vi "Traverse_Space_for new collision code.vi"(7 "Simulate/Run":T1=enum."Run VI", 9 "Show Panel?":bool, 10 "Traverse Setup":string) -> (3 "Error Comments":string)   [LabVIEW 2022 SP3]
doc: "This is an example of using features of the VI Server as a client. It shows how you might browse from one or more applications that may be exporting data from one or more data stations. \n\nThe example shows how to query a server for its list of exported VIs, how to get references to the VIs, and how call them with the Call By Reference function."
uses:
  Route mapping/Box_size.ctl
  Controls/ok_button.ctl
  Controls/User_Specific_mode.ctl
  Collision_Detection/Triangles/EnFlo specific/Collision Detection global.vi
  Globals/Constants_global.vi
  Globals/Trav_pos_global.vi
  Globals/Preference_global.vi
  Route mapping/Route_mapping_global.vi
panel:
  in  "Fixed Objects Name":u16(ring) items=["BeamCheck_Box_16500", "None"]
  out "Message":string
  in  "Probe Support":T2=[{"Max"=15001.0, "Min"=12000.0}, {"Max"=1000.0, "Min"=-1000.0}, {"Max"=700.0, "Min"=0.0}] {"Min" format="%#.1f"; "Max" format="%#.1f"}
  out "XYZ string":string
  out "XY string":string
  out "X string":string
  in  "X Component":u16(ring) items=["EnFlo_Trav1_X - Copy.stl", "EnFlo_Trav1_X.stl", "EnFlo_Trav1_X_original.stl", "Hello.stl", "None.stl"]
  in  "XYZ Component (Measurement Probe)":u16(ring) items=["None", "XYZ_20190131", "XYZ_20190918"]
  in  "XY Component (Traverse Boom)":u16(ring) items=["EnFlo_Trav1_XY.stl", "EnFlo_Trav1_XY_Long.stl", "EnFlo_Trav1_XY_Long_UW_laydown.stl", "EnFlo_Trav1_XY_Long_X400mm.stl", "EnFlo_Trav1_XY_Medium.stl", "EnFlo_Trav1_XY_Medium_FFID.stl", "EnFlo_Trav1_XY_Medium_UV_vertical.stl", "EnFlo_Trav1_XY_Medium_UW_laydown.stl", "None.stl"]
  in  "Model Name":u16(ring) items=["DIPLOS_array", "DIPLOS_array_0", "DIPLOS_array_45", "DSTL_Dapple_46", "Elysee", "Elysee_original", "Elysee_Source1", "Elysee_Source2", "Elysee_Source3", "MAGIC_1to500_Extra_8SE", "MAGIC_1to500_plus8", "MAGIC_1to500_plus8_fs", "MAGIC_London_Southbank_0_deg - Copy", "MAGIC_London_Southbank_0_deg _Case2", "MAGIC_London_Southbank_0_deg", "MAGIC_London_Southbank_0_deg_1to500", "MAGIC_London_Southbank_0_deg_1to500_without8SE", "MAGIC_London_Southbank_0_deg_21-08-19", "MAGIC_London_Southbank_0_deg_5_roofs", "MAGIC_London_Southbank_0_deg_ALL_roofs", "MAGIC_London_Southbank_0_deg_ALL_roofs_excl_bld12", "MAGIC_London_Southbank_0_deg_excl_12_and_150", "MAGIC_London_Southbank_0_deg_increasedHeights", "MAGIC_London_Southbank_0_deg_plus8", "MAGIC_London_Southbank_0_deg_plus8_bldg139roofblocks", "MAGIC_London_Southbank_0_deg_roofs", "MAGIC_London_Southbank_0_deg_roofs_3,8,10,49,60", "MAGIC_London_Southbank_0_deg_st8", "MAGIC_London_Southbank_VerMarco", "MAGIC_mic01_0_deg", "None", "Simple_C", "Simple_V", "Single_Cube_H240", "Single_Tall_Bldg"]
  in  "Traverse Name":u16(ring) items=["EnFlo_Stack", "EnFlo_Trav1", "EnFlo_Trav3", "EnFlo_Trav4", "EnFlo_Tunnel", "EnFlo_Turntable", "Laser_Disp_Scanner"]
  in  "Cancel Button":bool
  in  "OK":T3
  in  "Traverse Limits":T2=[{"Max"=15001.0, "Min"=12000.0}, {"Max"=1000.0, "Min"=-1000.0}, {"Max"=700.0, "Min"=0.0}] {"Min" format="%#.1f"; "Max" format="%#.1f"}
  # "Enter all coordinates assuming the Model Orientation is zero degrees"
  # "X                           Y                          Z"
  # "All geometry always reloaded after running this panel"
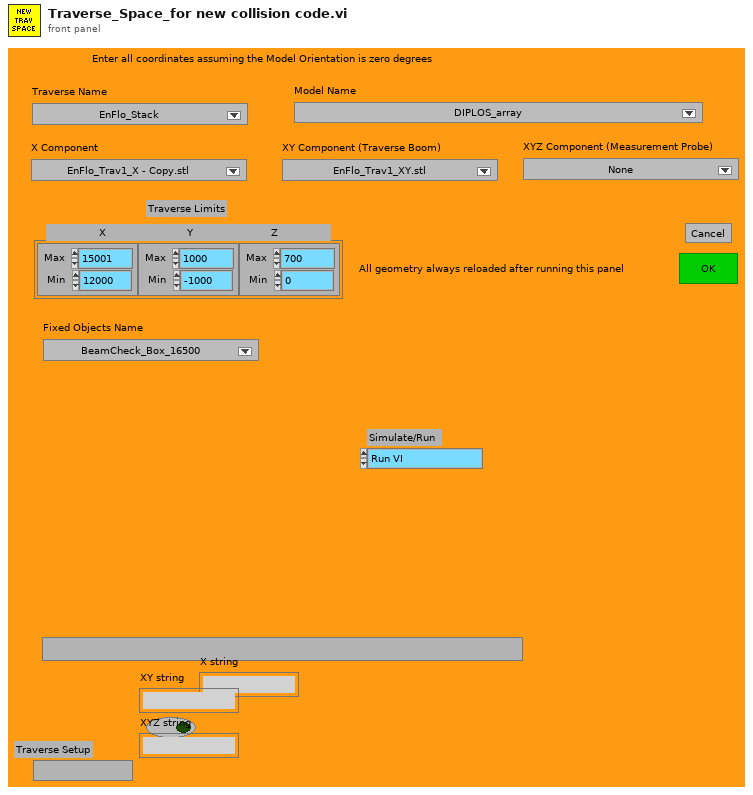
[diagram p1: front panel]
types:
  T1 = typedef "User_Specific_mode.ctl" = enum16{"Check VI only", "Run VI"}
  T2 = typedef "Box_size.ctl" = cluster{"Max":sgl, "Min":sgl}[]
  T3 = typedef "ok_button.ctl" = bool
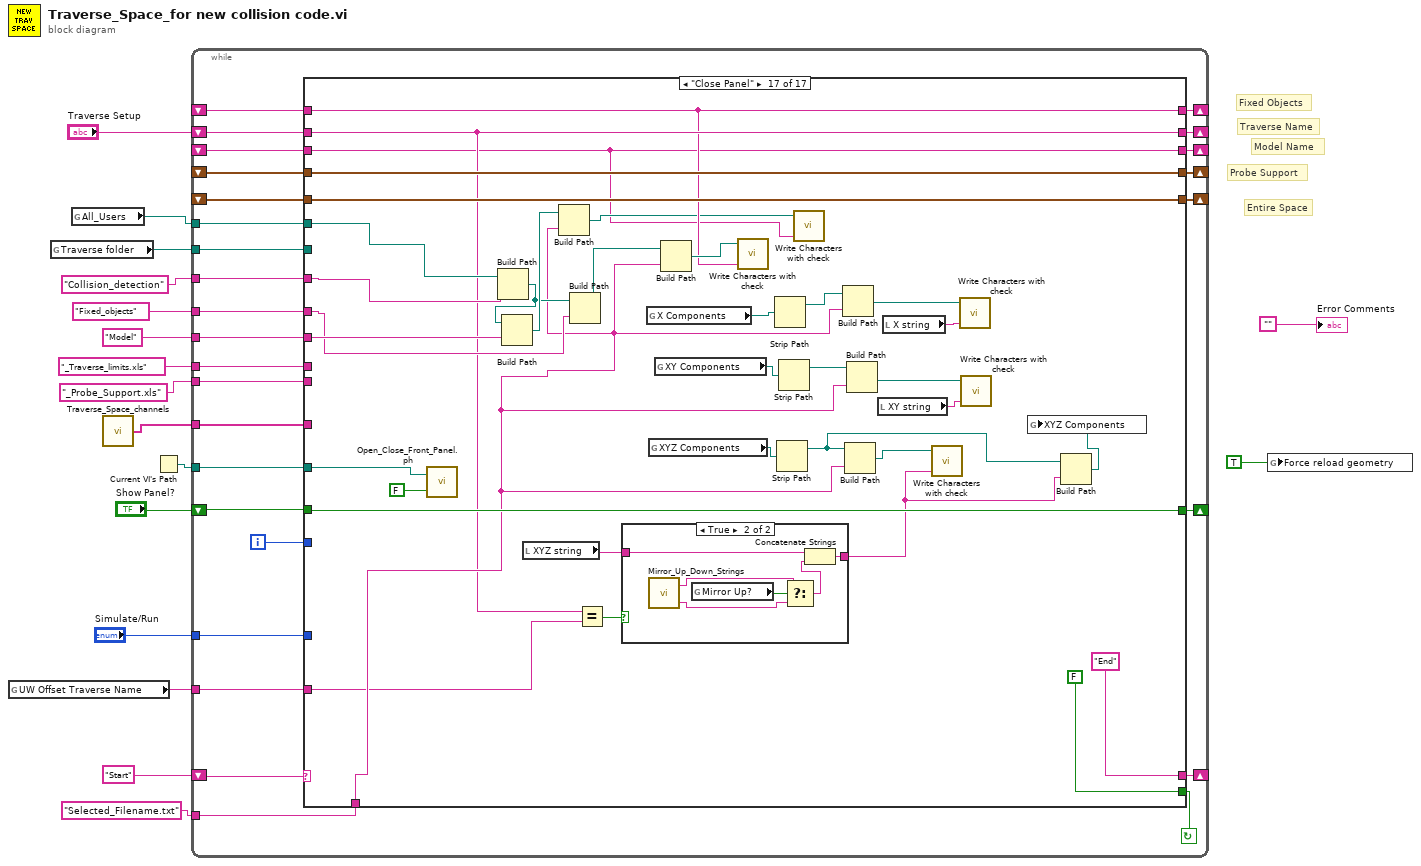
[diagram p0: block diagram]
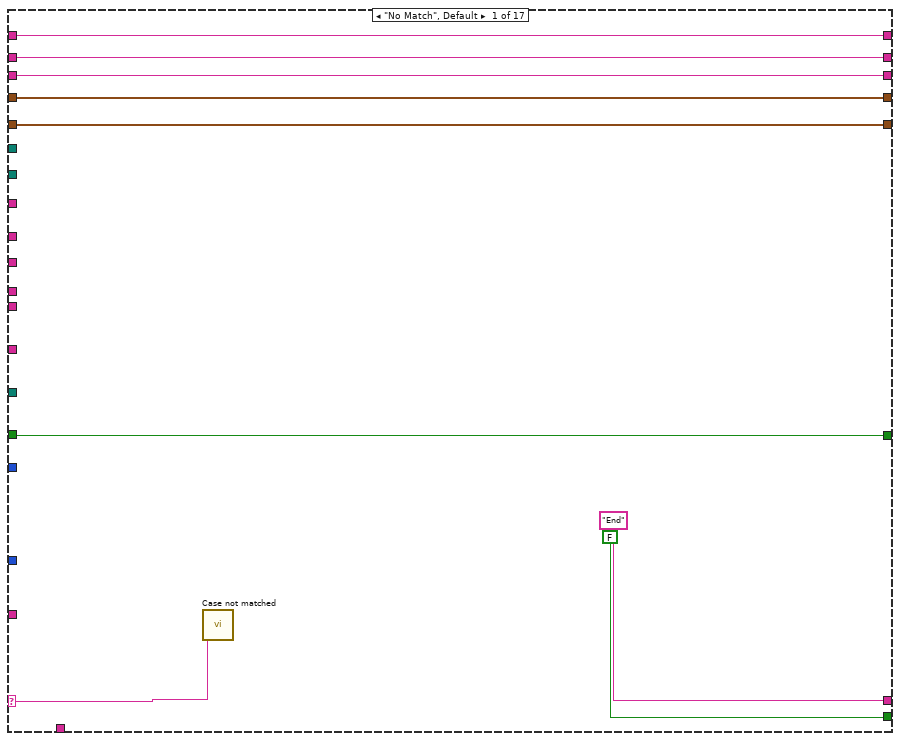
[diagram p2: hidden frame]
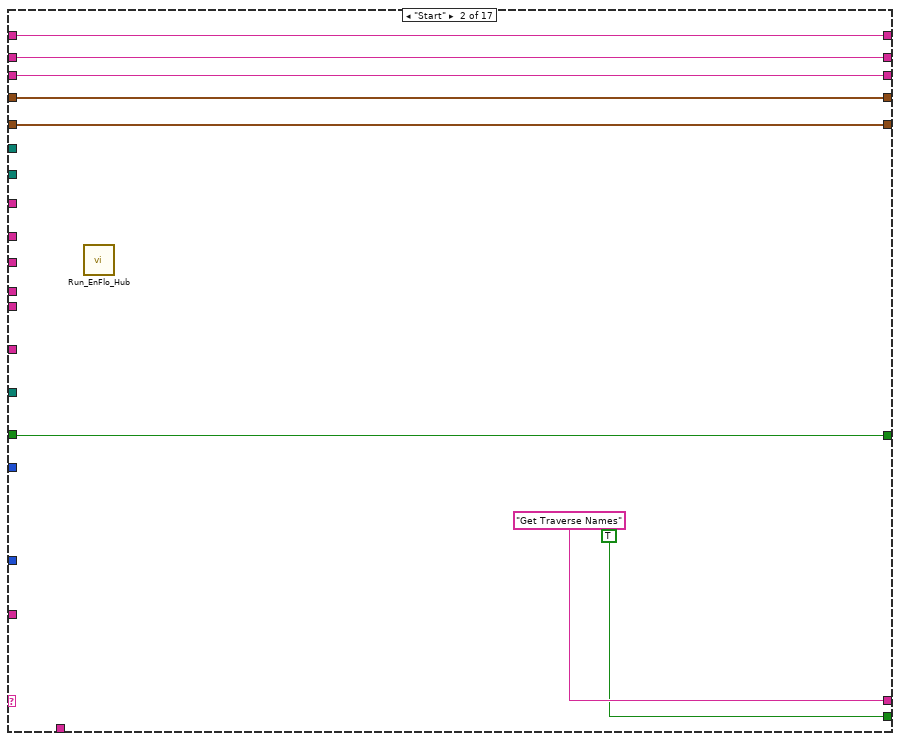
[diagram p3: hidden frame]
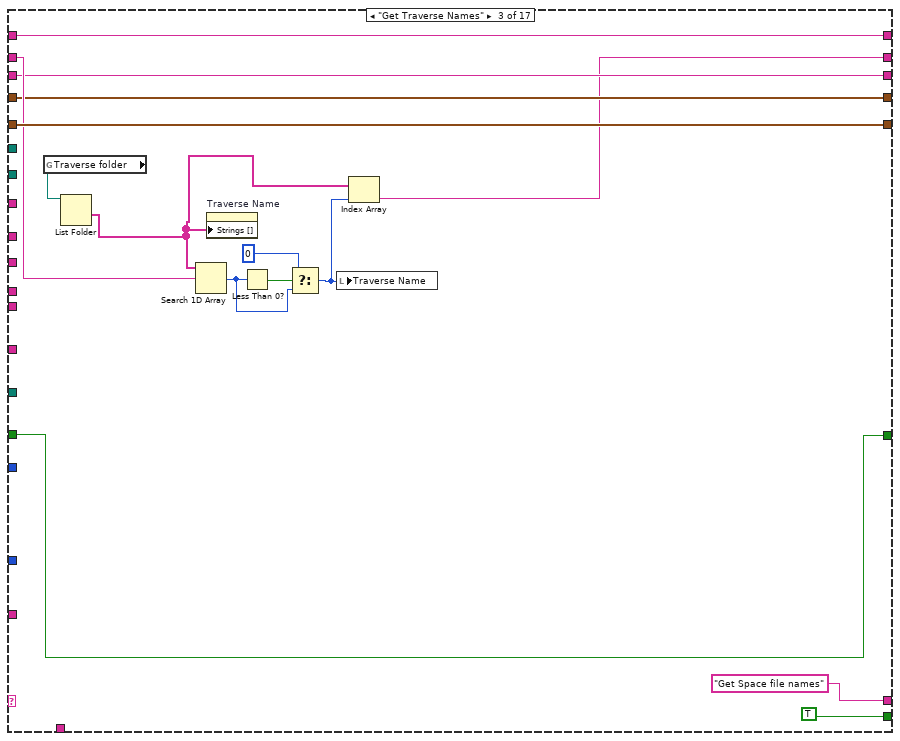
[diagram p4: hidden frame]
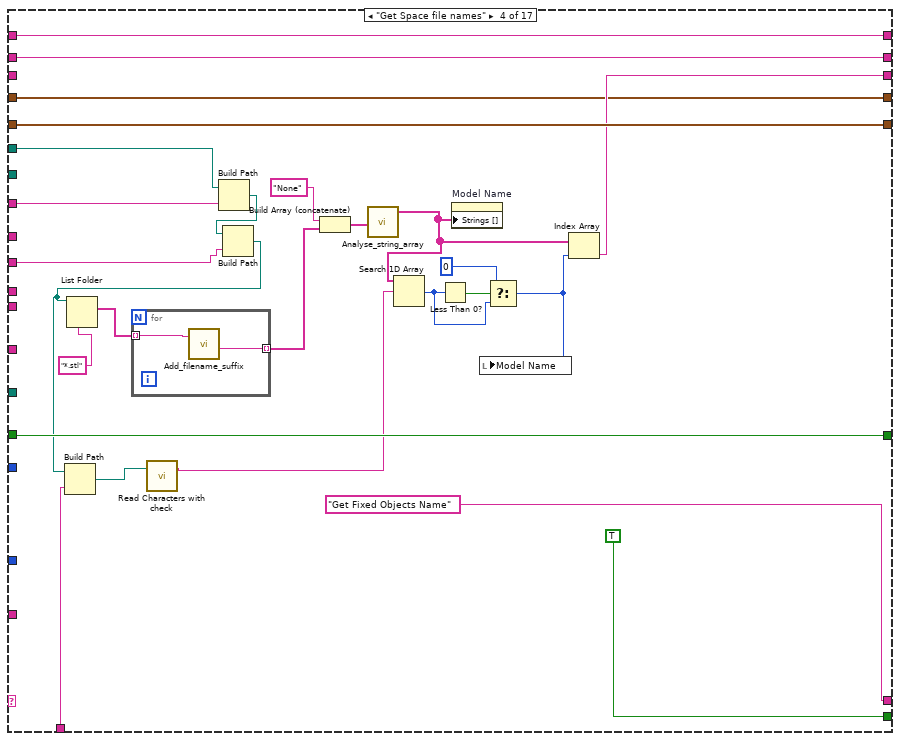
[diagram p5: hidden frame]
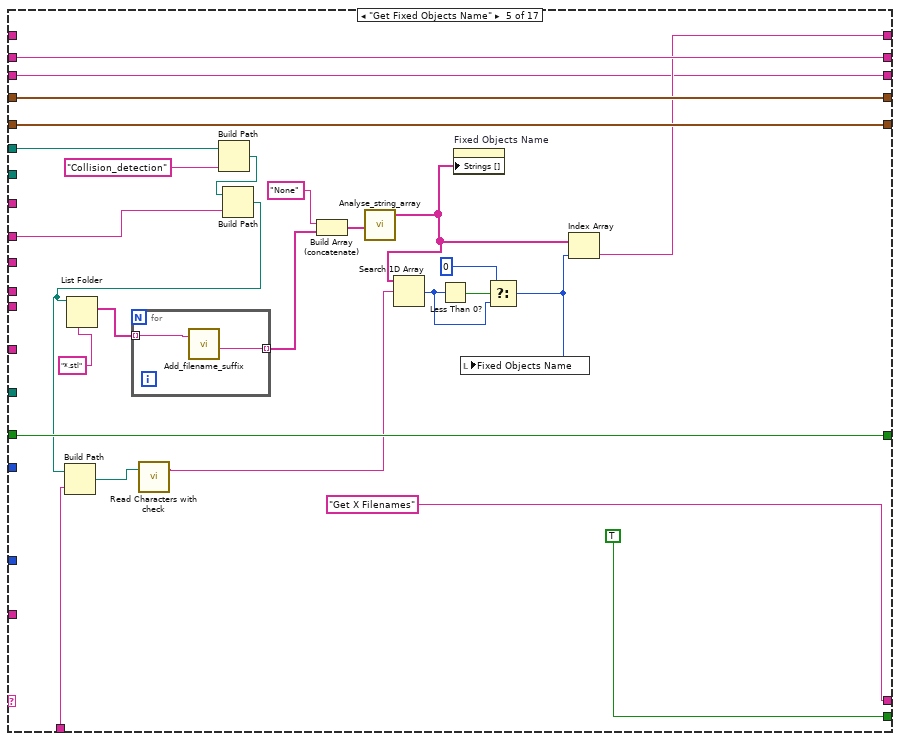
[diagram p6: hidden frame]
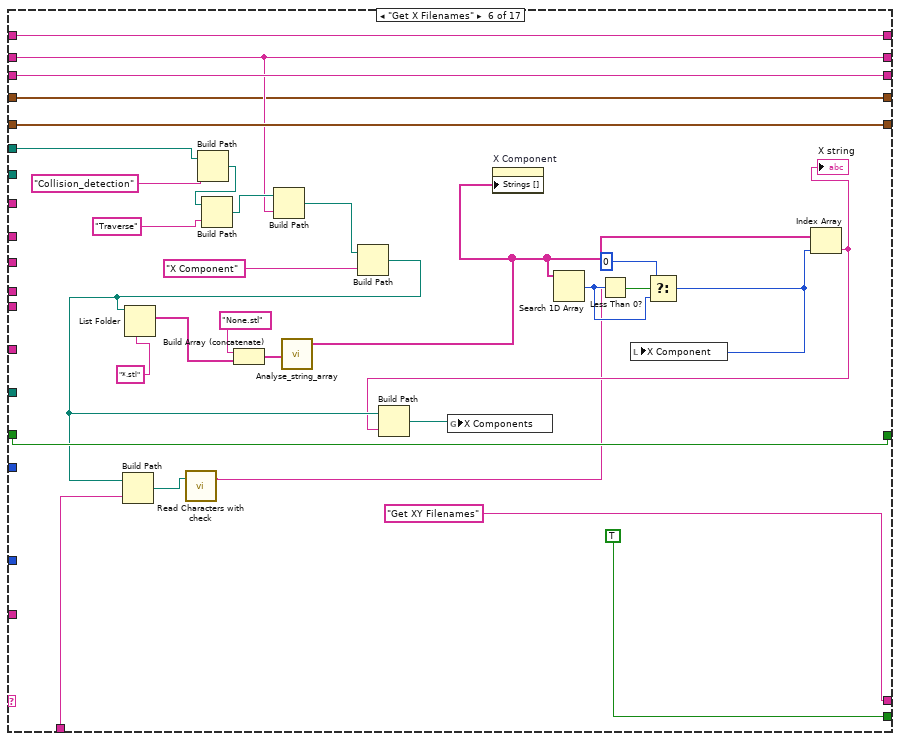
[diagram p7: hidden frame]
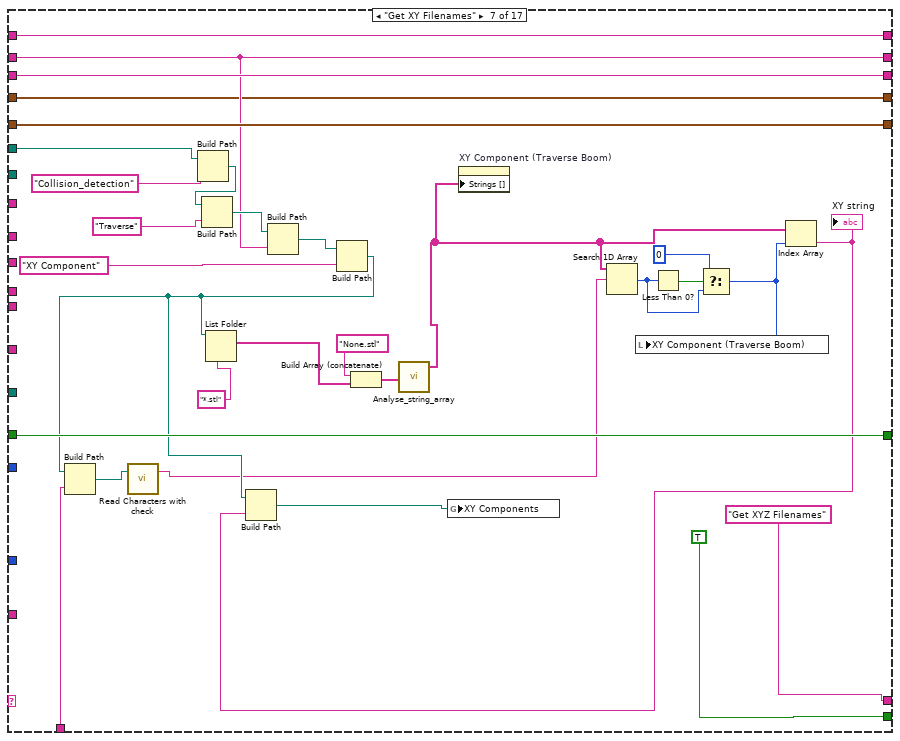
[diagram p8: hidden frame]
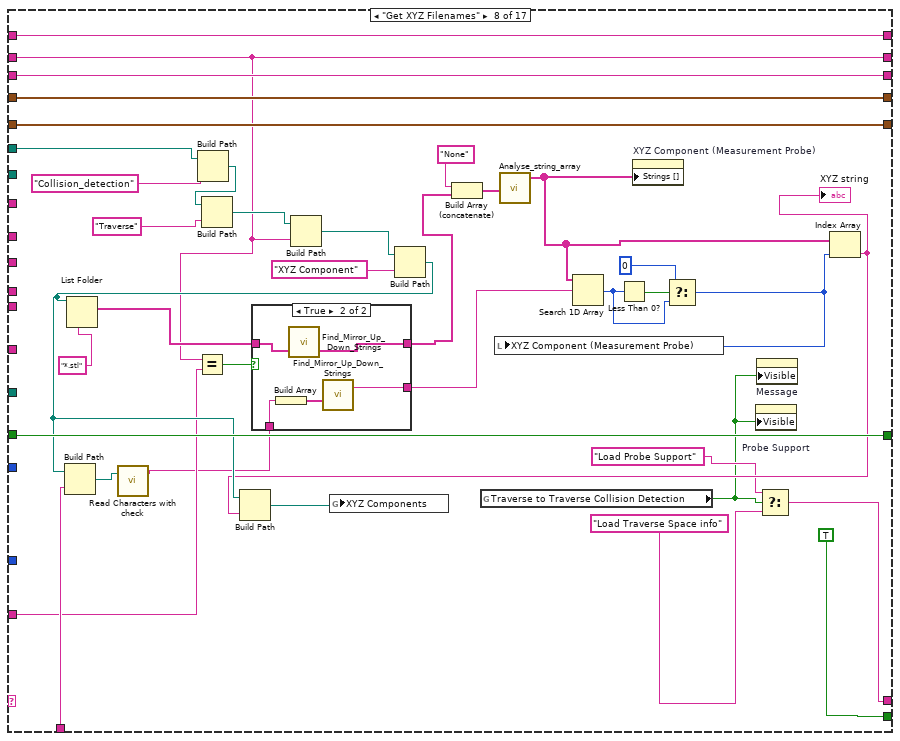
[diagram p9: hidden frame]
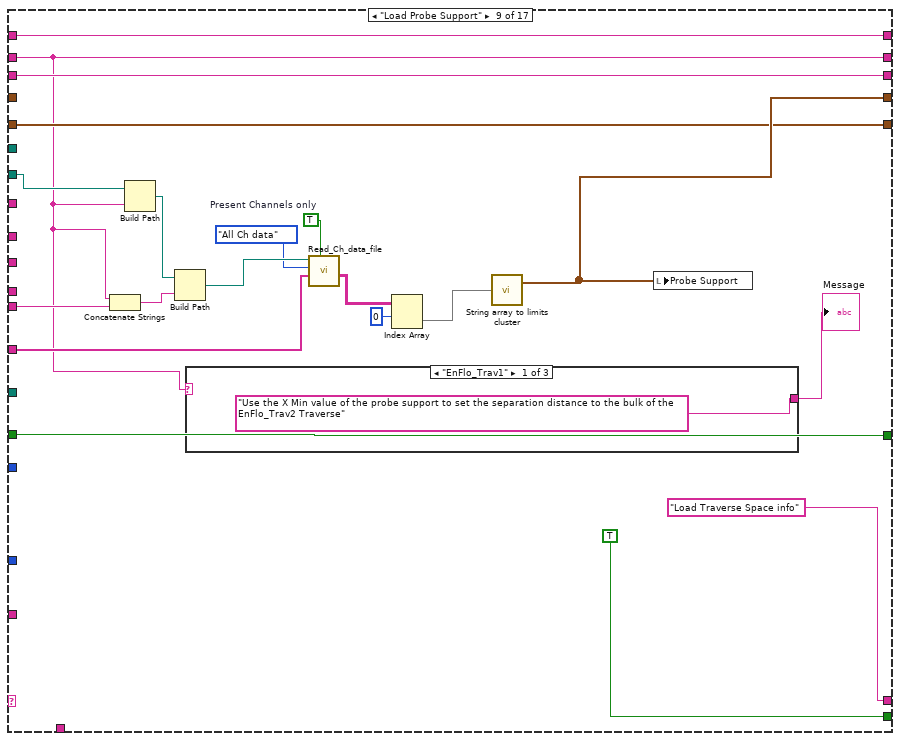
[diagram p11: hidden frame]
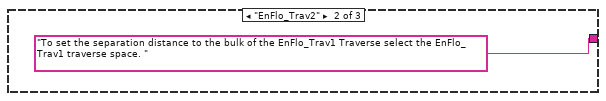
[diagram p12: hidden frame]
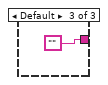
[diagram p13: hidden frame]
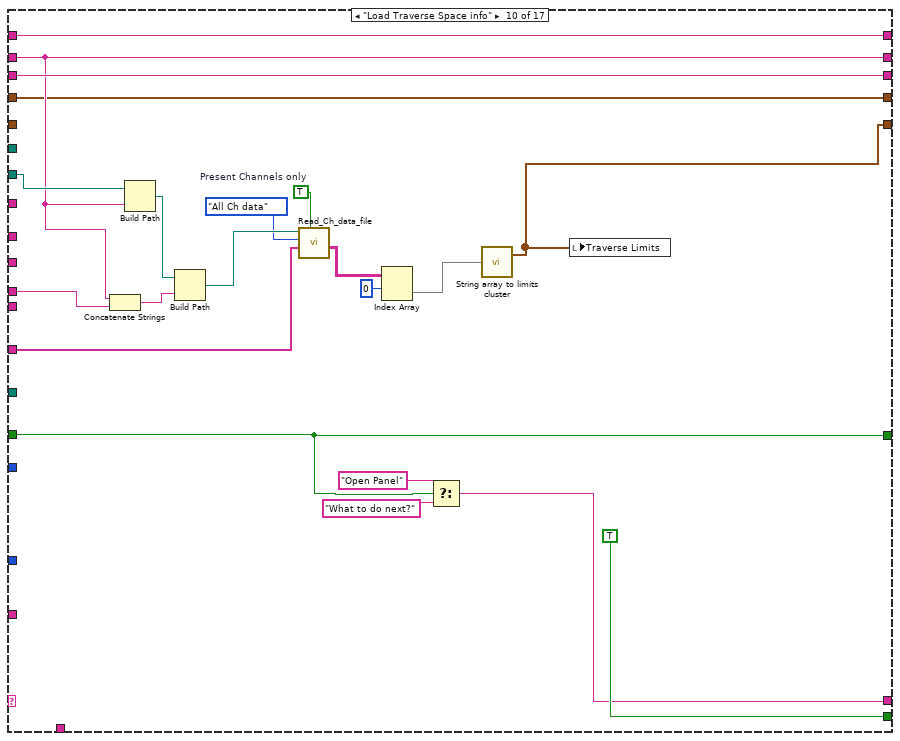
[diagram p14: hidden frame]
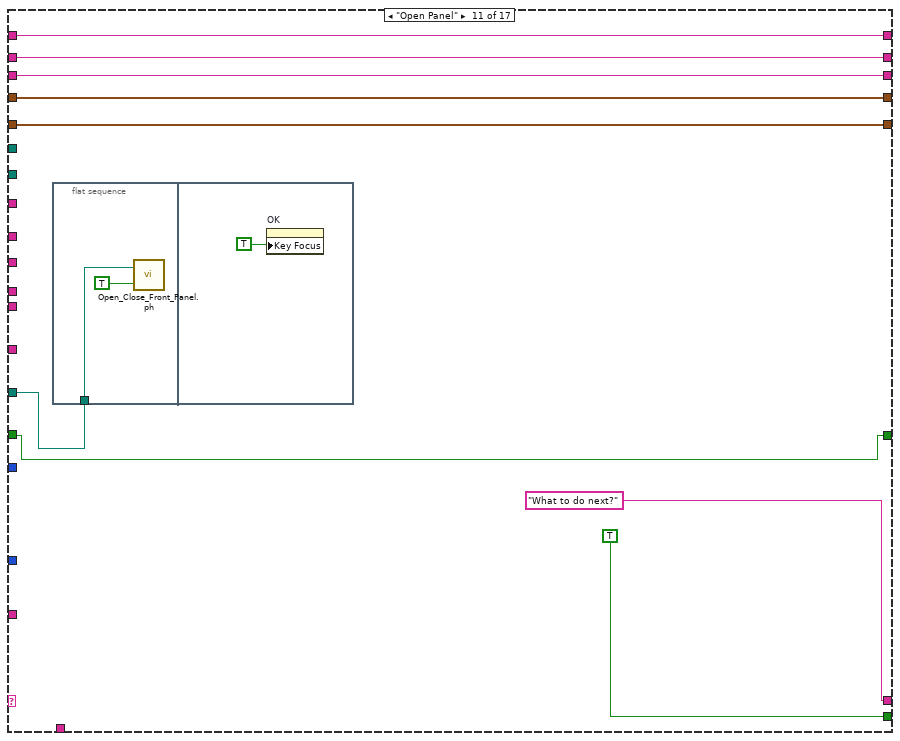
[diagram p15: hidden frame]
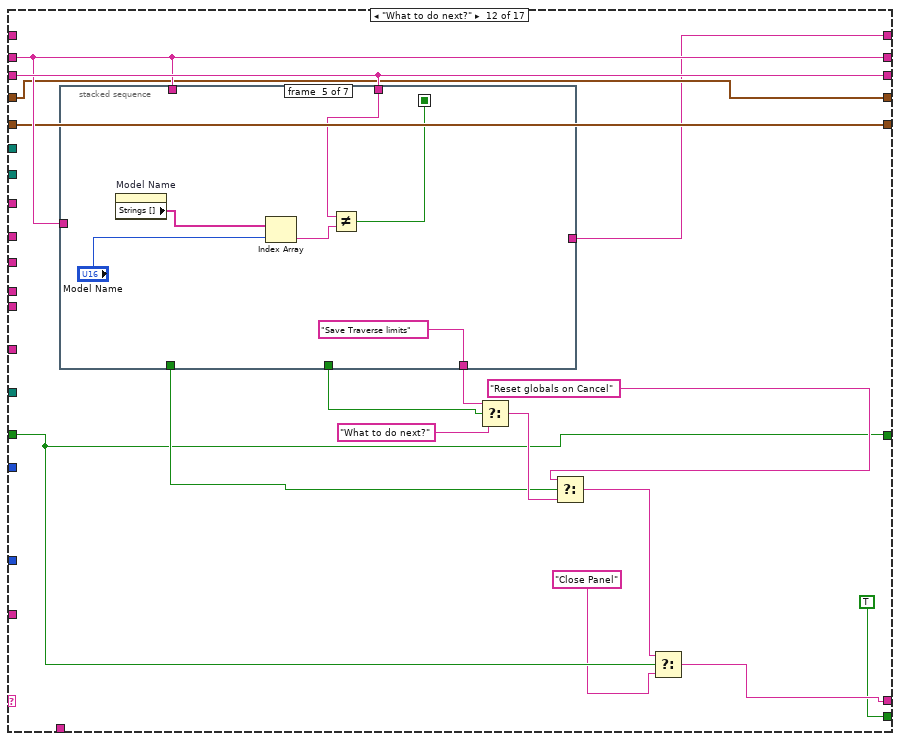
[diagram p16: hidden frame]
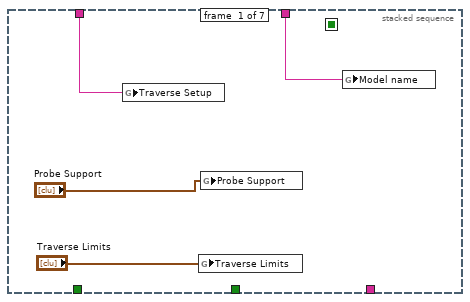
[diagram p17: hidden frame]
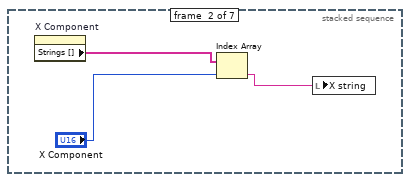
[diagram p18: hidden frame]
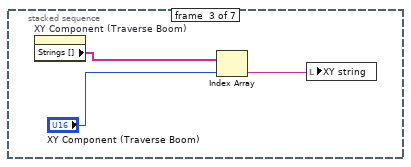
[diagram p19: hidden frame]
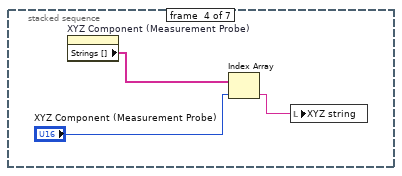
[diagram p20: hidden frame]
diagram:
  # "Fixed Objects"
  # "Probe Support"
  # "Traverse Name"
  # "Model Name"
  # "Entire Space"
  n1 = global read "Trav_pos_global.vi" "UW Offset Traverse Name"() -> (w1:string)
  n2 = global read "Constants_global.vi" "Traverse folder"() -> (w13:path)
  n3 = global read "Constants_global.vi" "All_Users"() -> (w10:path)
  n4 = call "Traverse_Space_channels.vi"() -> ("Channel Names"=w11:string[])
  n5 = Current VI's Path() -> (path=w16:path)
  n6 = while {
    shift-left: "Start" -> [w41]
    shift-right: [w43] -> _
    tunnel: w16 -> [w42]
    shift-right: [w40] -> _
    shift-left: _ -> [w39]
    shift-right: [w37] -> _
    shift-left: "Traverse Setup" -> [w35]
    shift-right: [w38] -> _
    shift-left: _ -> [w36]
    shift-right: [w33] -> _
    shift-left: "Show Panel?" -> [w34]
    tunnel: w13 -> [w32]
    tunnel: "_Traverse_limits.xls" ("string") -> [w31]
    tunnel: w11 -> [w30]
    tunnel: w10 -> [w29]
    tunnel: "Selected_Filename.txt" ("Substring") -> [w28]
    tunnel: "_Probe_Support.xls" ("string") -> [w27]
    shift-right: [w25] -> _
    shift-left: _ -> [w26]
    shift-right: [w24] -> _
    shift-left: _ -> [w23]
    tunnel: "Model" ("Substring") -> [w22]
    tunnel: "Collision_detection" ("Substring") -> [w21]
    tunnel: "Fixed_objects" ("Substring") -> [w20]
    tunnel: "Simulate/Run" -> [w19]
    tunnel: w1 -> [w18]
    i -> [w45]
    stop <- w44 continue-if-true
    n7 = case shown="\"Close Panel\"" w41 {
      tunnel: w45 -> [_ _ _ _ _ _ _ _ _ _ _ _ _ _ _ _ _]
      tunnel: [FALSE ("status") TRUE ("status") TRUE ("status") TRUE ("status") TRUE ("status") TRUE ("status") TRUE ("status") TRUE ("status") TRUE ("status") TRUE ("status") TRUE ("status") TRUE ("status") TRUE ("status") TRUE ("status") w411 TRUE ("status") FALSE ("status")] -> w44
      selector: w41 -> [w46 _ _ _ _ _ _ _ _ _ _ _ _ _ _ _ _]
      tunnel: ["End" ("f") "Get Traverse Names" ("f") "Get Space file names" ("f") "Get Fixed Objects Name" "Get X Filenames" "Get XY Filenames" "Get XYZ Filenames" w210 "Load Traverse Space info" w280 "What to do next?" w296 "Save Probe Support info" "Load another space file?" w412 "Close Panel" "End"] -> w43
      tunnel: w34 -> [w49 w57 w68 w94 w122 w155 w185 w224 w247 w266 w284 w299 w350 w384 w411 w442 w476]
      tunnel: w42 -> [_ _ _ _ _ _ _ _ _ _ w287 _ _ _ _ _ w478]
      tunnel: [w52 w62 w76 w101 w129 w161 w191 w229 w241 w269 w288 w301 w353 w387 w417 w444 w477] -> w40
      tunnel: w39 -> [w52 w62 w76 w101 w129 w161 w191 w229 w241 _ w288 w301 w353 w387 w417 w444 w477]
      tunnel: [w50 w58 w67 w96 w113 w148 w178 w217 w256 w277 w285 w305 w351 w385 w413 w440 w446] -> w38
      tunnel: [w51 w59 w63 w95 w123 w146 w176 w201 w239 w264 w286 w302 w348 w383 w415 w441 w456] -> w37
      tunnel: w36 -> [w50 w58 w67 _ w113 w148 w178 w217 w256 w277 w285 w305 w351 w385 w414 w440 w446]
      tunnel: w35 -> [w51 w59 w71 w95 w123 w146 w176 w201 w239 w264 w286 w302 w348 w383 w416 w441 w456]
      tunnel: [w49 w57 w68 w94 w122 w155 w185 w224 w247 w266 w284 w299 w350 w384 w411 w442 w476] -> w33
      tunnel: w32 -> [_ _ _ _ _ _ _ _ w246 w265 _ _ w347 w382 _ _ _]
      tunnel: w31 -> [_ _ _ _ _ _ _ _ _ w268 _ _ w346 _ _ _ _]
      tunnel: w30 -> [_ _ _ _ _ _ _ _ w248 w267 _ _ w345 w381 _ _ _]
      tunnel: w29 -> [_ _ _ w90 w118 w151 w181 w220 _ _ _ _ _ _ _ _ w474]
      tunnel: w28 -> [_ _ _ w89 w117 w150 w180 w219 _ _ _ _ _ _ _ _ w459]
      tunnel: w27 -> [_ _ _ _ _ _ _ _ w243 _ _ _ _ w377 _ _ _]
      tunnel: [w48 w56 w66 w87 w115 w141 w171 w207 w242 w262 w283 w300 w349 w376 w410 w439 w468] -> w25
      tunnel: w26 -> [w48 w56 w66 w87 w115 w141 w171 w207 _ w262 w283 w300 w349 w376 w410 w439 w468]
      tunnel: [w47 w55 w65 w86 w114 w140 w170 w204 w238 w261 w282 w294 w341 w375 w409 w438 w454] -> w24
      tunnel: w23 -> [w47 w55 w65 w86 _ w140 w170 w204 w238 w261 w282 _ w341 w375 w409 w438 w454]
      tunnel: w22 -> [_ _ _ w85 _ _ _ _ _ _ _ _ _ _ _ _ w464]
      tunnel: w21 -> [_ _ _ w84 _ _ _ _ _ _ _ _ _ _ _ _ w463]
      tunnel: w20 -> [_ _ _ _ w112 _ _ _ _ _ _ _ _ _ _ _ w461]
      tunnel: w19 -> [_ _ _ _ _ _ _ _ _ _ _ _ _ _ _ _ _]
      tunnel: w18 -> [_ _ _ _ _ _ _ w202 _ _ _ _ _ _ _ _ w457]
      frame "No Match", Default {
        n8 = call "Case not matched.vi"("Case Name not Matched"=w46) -> ()
      }
      frame "Start" {
        n9 = call "Run_EnFlo_Hub.vi"() -> ()  [unwired: 1 in, 7 out]
      }
      frame "Get Traverse Names" {
        n10 = global read "Constants_global.vi" "Traverse folder"() -> (w70:path)
        n11 = List Folder(path=w70) -> (folder names=w69:string[])  [unwired: 1 in, 5 out]
        n12 = Search 1D Array(1D array=w69, element=w71) -> (index of element=w74:i32)  [unwired: 1 out]
        n13 = property on="Traverse Name" class="Ring (strict)"("Strings []"=w69) -> ()  [unwired: 2 in, 2 out]
        n14 = Less Than 0?(x=w74) -> (x < 0?=w75:bool)
        n15 = Select(t=0, s=w75, f=w74) -> (s? t:f=w72:i32)
        n16 = local write "Traverse Name"(w72) -> ()
        n17 = Index Array(array=w69, index=w72) -> (element=w63:string)
      }
      frame "Get Space file names" {
        n18 = Build Path(base path=w90, name or relative path=w84) -> (appended path=w93:path)
        n19 = Build Path(base path=w93, name or relative path=w85) -> (appended path=w91:path)
        n20 = Build Path(base path=w91, name or relative path=w89) -> (appended path=w79:path)
        n21 = List Folder(path=w91, pattern="*.stl") -> (filenames=w88:string[])  [unwired: 1 in, 4 out]
        n22 = for {
          tunnel: w88 -> [w105] mode=indexing
          tunnel: [w104] -> w83 mode=indexing
          n23 = call "Add_filename_suffix.vi"("Filename"=w105) -> ("Base name"=w104:string)  [unwired: 1 in, 3 out]
        }
        n24 = call "Read Characters with check.vi"("file (use dialog)"=w79) -> ("Read String"=w78:string)  [unwired: 1 in, 1 out]
        n25 = Build Array (concatenate)("None", w83) -> (w81:string[])
        n26 = call "Analyse_string_array.vi"("String array"=w81) -> ("Unique strings"=w80:string[])  [unwired: 1 in, 1 out]
        n27 = Search 1D Array(1D array=w80, element=w78) -> (index of element=w99:i32)  [unwired: 1 out]
        n28 = Less Than 0?(x=w99) -> (x < 0?=w100:bool)
        n29 = property on="Model Name" class="Ring (strict)"("Strings []"=w80) -> ()  [unwired: 2 in, 2 out]
        n30 = Select(t=0, s=w100, f=w99) -> (s? t:f=w97:i32)
        n31 = local write "Model Name"(w97) -> ()
        n32 = Index Array(array=w80, index=w97) -> (element=w96:string)
      }
      frame "Get Fixed Objects Name" {
        n33 = Build Path(base path=w118, name or relative path="Collision_detection" ("Substring")) -> (appended path=w121:path)
        n34 = Build Path(base path=w121, name or relative path=w112) -> (appended path=w119:path)
        n35 = Build Path(base path=w119, name or relative path=w117) -> (appended path=w107:path)
        n36 = List Folder(path=w119, pattern="*.stl") -> (filenames=w116:string[])  [unwired: 1 in, 4 out]
        n37 = for {
          tunnel: w116 -> [w133] mode=indexing
          tunnel: [w132] -> w109 mode=indexing
          n38 = call "Add_filename_suffix.vi"("Filename"=w133) -> ("Base name"=w132:string)  [unwired: 1 in, 3 out]
        }
        n39 = call "Read Characters with check.vi"("file (use dialog)"=w107) -> ("Read String"=w106:string)  [unwired: 1 in, 1 out]
        n40 = Build Array (concatenate)("None", w109) -> (w110:string[])
        n41 = call "Analyse_string_array.vi"("String array"=w110) -> ("Unique strings"=w108:string[])  [unwired: 1 in, 1 out]
        n42 = Search 1D Array(1D array=w108, element=w106) -> (index of element=w127:i32)  [unwired: 1 out]
        n43 = Less Than 0?(x=w127) -> (x < 0?=w128:bool)
        n44 = property on="Fixed Objects Name" class="Ring (strict)"("Strings []"=w108) -> ()  [unwired: 2 in, 2 out]
        n45 = Select(t=0, s=w128, f=w127) -> (s? t:f=w124:i32)
        n46 = local write "Fixed Objects Name"(w124) -> ()
        n47 = Index Array(array=w108, index=w124) -> (element=w114:string)
      }
      frame "Get X Filenames" {
        n48 = Build Path(base path=w151, name or relative path="Collision_detection" ("Substring")) -> (appended path=w154:path)
        n49 = Build Path(base path=w154, name or relative path="Traverse" ("Substring")) -> (appended path=w147:path)
        n50 = Build Path(base path=w147, name or relative path=w146) -> (appended path=w145:path)
        n51 = Build Path(base path=w145, name or relative path="X Component") -> (appended path=w144:path)
        n52 = Build Path(base path=w144, name or relative path=w150) -> (appended path=w135:path)
        n53 = List Folder(path=w144, pattern="*.stl") -> (filenames=w137:string[])  [unwired: 1 in, 4 out]
        n54 = call "Read Characters with check.vi"("file (use dialog)"=w135) -> ("Read String"=w134:string)  [unwired: 1 in, 1 out]
        n55 = Build Array (concatenate)("None.stl", w137) -> (w138:string[])
        n56 = call "Analyse_string_array.vi"("String array"=w138) -> ("Unique strings"=w136:string[])  [unwired: 1 in, 1 out]
        n57 = property on="X Component" class="Ring (strict)"("Strings []"=w136) -> ()  [unwired: 2 in, 2 out]
        n58 = Search 1D Array(1D array=w136, element=w134) -> (index of element=w159:i32)  [unwired: 1 out]
        n59 = Less Than 0?(x=w159) -> (x < 0?=w160:bool)
        n60 = Select(t=0, s=w160, f=w159) -> (s? t:f=w156:i32)
        n61 = local write "X Component"(w156) -> ()
        n62 = Index Array(array=w136, index=w156) -> (element=w143:string)
        "X string" <- w143
        n63 = Build Path(base path=w144, name or relative path=w143) -> (appended path=w142:path)
        n64 = global write "Collision Detection global.vi" "X Components"(w142) -> ()
      }
      frame "Get XY Filenames" {
        n65 = Build Path(base path=w181, name or relative path="Collision_detection" ("Substring")) -> (appended path=w184:path)
        n66 = Build Path(base path=w184, name or relative path="Traverse" ("Substring")) -> (appended path=w177:path)
        n67 = Build Path(base path=w177, name or relative path=w176) -> (appended path=w175:path)
        n68 = Build Path(base path=w175, name or relative path="XY Component") -> (appended path=w174:path)
        n69 = Build Path(base path=w174, name or relative path=w180) -> (appended path=w165:path)
        n70 = call "Read Characters with check.vi"("file (use dialog)"=w165) -> ("Read String"=w164:string)  [unwired: 1 in, 1 out]
        n71 = List Folder(path=w174, pattern="*.stl") -> (filenames=w167:string[])  [unwired: 1 in, 4 out]
        n72 = Build Array (concatenate)("None.stl", w167) -> (w168:string[])
        n73 = call "Analyse_string_array.vi"("String array"=w168) -> ("Unique strings"=w166:string[])  [unwired: 1 in, 1 out]
        n74 = property on="XY Component (Traverse Boom)" class="Ring (strict)"("Strings []"=w166) -> ()  [unwired: 2 in, 2 out]
        n75 = Search 1D Array(1D array=w166, element=w164) -> (index of element=w189:i32)  [unwired: 1 out]
        n76 = Less Than 0?(x=w189) -> (x < 0?=w190:bool)
        n77 = Select(t=0, s=w190, f=w189) -> (s? t:f=w186:i32)
        n78 = local write "XY Component (Traverse Boom)"(w186) -> ()
        n79 = Index Array(array=w166, index=w186) -> (element=w173:string)
        "XY string" <- w173
        n80 = Build Path(base path=w174, name or relative path=w173) -> (appended path=w172:path)
        n81 = global write "Collision Detection global.vi" "XY Components"(w172) -> ()
      }
      frame "Get XYZ Filenames" {
        n82 = Equal?(x=w201, y=w202) -> (x = y?=w200:bool)
        n83 = Build Path(base path=w220, name or relative path="Collision_detection" ("Substring")) -> (appended path=w223:path)
        n84 = Build Path(base path=w223, name or relative path="Traverse" ("Substring")) -> (appended path=w215:path)
        n85 = Build Path(base path=w215, name or relative path=w201) -> (appended path=w214:path)
        n86 = Build Path(base path=w214, name or relative path="XYZ Component") -> (appended path=w213:path)
        n87 = Build Path(base path=w213, name or relative path=w219) -> (appended path=w195:path)
        n88 = List Folder(path=w213, pattern="*.stl") -> (filenames=w205:string[])  [unwired: 1 in, 4 out]
        n89 = call "Read Characters with check.vi"("file (use dialog)"=w195) -> ("Read String"=w194:string)  [unwired: 1 in, 1 out]
        n90 = case shown="True" w200 {
          tunnel: w205 -> [w232 w237]
          tunnel: [w232 w236] -> w197
          tunnel: w194 -> [w231 w235]
          tunnel: [w231 w233] -> w203
          frame False {
          }
          frame True {
            n91 = Build Array(w235) -> (w234:string[])
            n92 = call "Find_Mirror_Up_Down_Strings.vi"("Filenames"=w237) -> ("Base Filenames to display"=w236:string[])  [unwired: 1 in, 1 out]
            n93 = call "Find_Mirror_Up_Down_Strings.vi"("Filenames"=w234) -> ("1st Basename"=w233:string)  [unwired: 1 in, 1 out]
          }
        }
        n94 = Build Array (concatenate)("None", w197) -> (w198:string[])
        n95 = global read "Preference_global.vi" "Traverse to Traverse Collision Detection"() -> (w206:bool)
        n96 = call "Analyse_string_array.vi"("String array"=w198) -> ("Unique strings"=w196:string[])  [unwired: 1 in, 1 out]
        n97 = Search 1D Array(1D array=w196, element=w203) -> (index of element=w227:i32)  [unwired: 1 out]
        n98 = Less Than 0?(x=w227) -> (x < 0?=w228:bool)
        n99 = property on="XYZ Component (Measurement Probe)" class="Ring (strict)"("Strings []"=w196) -> ()  [unwired: 2 in, 2 out]
        n100 = Select(t=0, s=w228, f=w227) -> (s? t:f=w216:i32)
        n101 = local write "XYZ Component (Measurement Probe)"(w216) -> ()
        n102 = property on="Probe Support" class="Arr (strict)"("Visible"=w206) -> ()  [unwired: 2 in, 2 out]
        n103 = property on="Message" class="Str"("Visible"=w206) -> ()  [unwired: 2 in, 2 out]
        n104 = Select(t="Load Probe Support", s=w206, f="Load Traverse Space info") -> (s? t:f=w210:string)
        n105 = Index Array(array=w196, index=w216) -> (element=w212:string)
        "XYZ string" <- w212
        n106 = Build Path(base path=w213, name or relative path=w212) -> (appended path=w211:path)
        n107 = global write "Collision Detection global.vi" "XYZ Components"(w211) -> ()
      }
      frame "Load Probe Support" {
        w250 = TRUE  # Present Channels only
        n108 = Concatenate Strings(w239, w243) -> (w251:string)
        n109 = Build Path(base path=w246, name or relative path=w239) -> (appended path=w245:path)
        n110 = Build Path(base path=w245, name or relative path=w251) -> (appended path=w252:path)
        n111 = case shown="\"EnFlo_Trav1\"" w239 {
          tunnel: ["Use the X Min value of the probe support to set the separation distance to the bulk of the EnFlo_Trav2 Traverse" "To set the separation distance to the bulk of the EnFlo_Trav1 Traverse select the EnFlo_Trav1 traverse space. " ""] -> w240
          frame "EnFlo_Trav1" {
          }
          frame "EnFlo_Trav2" {
          }
          frame Default {
          }
        }
        "Message" <- w240
        n112 = call "Read_Ch_data_file.vi"("Present Channels only"=w250, "Present Channels"=w248, "Output"=enum16{"All Ch data", "The last few rows"}."All Ch data", "Filename"=w252) -> ("Channel Values"=w253:string[][])  [unwired: 1 in, 4 out]
        n113 = Index Array(array=w253, index (row)=0) -> (element=w255:string[])  [unwired: 1 in]
        n114 = call "String array to limits cluster.vi"("Channel Values in"=w255) -> ("Limits out"=w242:T2)  [unwired: 1 out]
        n115 = local write "Probe Support"(w242) -> ()
      }
      frame "Load Traverse Space info" {
        w271 = TRUE  # Present Channels only
        n116 = Concatenate Strings(w264, w268) -> (w272:string)
        n117 = Build Path(base path=w265, name or relative path=w264) -> (appended path=w263:path)
        n118 = Build Path(base path=w263, name or relative path=w272) -> (appended path=w273:path)
        n119 = call "Read_Ch_data_file.vi"("Present Channels only"=w271, "Present Channels"=w267, "Output"=enum16{"All Ch data", "The last few rows"}."All Ch data", "Filename"=w273) -> ("Channel Values"=w274:string[][])  [unwired: 1 in, 4 out]
        n120 = Index Array(array=w274, index (row)=0) -> (element=w276:string[])  [unwired: 1 in]
        n121 = Select(t="Open Panel", s=w266, f="What to do next?") -> (s? t:f=w280:string)
        n122 = call "String array to limits cluster.vi"("Channel Values in"=w276) -> ("Limits out"=w269:T2)  [unwired: 1 out]
        n123 = local write "Traverse Limits"(w269) -> ()
      }
      frame "Open Panel" {
        n124 = flat-sequence {
          tunnel: w287 -> [w291]
          frame #0 {
            n125 = call "Open_Close_Front_Panel.ph.vi"("openWindow (T)"=TRUE ("Front Panel Window:Open"), "VI path"=w291) -> ()  [unwired: 1 in, 1 out]
          }
          frame #1 {
            n126 = property on="OK" class="Bool"("Key Focus"=TRUE) -> ()  [unwired: 2 in, 2 out]
          }
        }
      }
      frame "What to do next?" {
        n127 = stacked-sequence {
          seq-local: [_ _ _ _ w324 _ _] -> [_ _ _ _ _ _ w332]
          tunnel: w302 -> [_ _ _ _ _ _ w337]
          tunnel: [_ _ _ _ _ _ w333] -> w307
          tunnel: [_ _ _ _ _ _ "Cancel Button"] -> w306
          tunnel: w305 -> [w312 _ _ _ w325 _ _]
          tunnel: [_ _ _ _ "Save Traverse limits" _ _] -> w303
          tunnel: w302 -> [w313 _ _ _ _ _ _]
          tunnel: [_ _ _ _ _ w329 _] -> w294
          frame #0 {
            n128 = global write "Route_mapping_global.vi" "Traverse Setup"(w313) -> ()
            n129 = global write "Route_mapping_global.vi" "Traverse Limits"("Traverse Limits") -> ()
            n130 = global write "Route_mapping_global.vi" "Probe Support"("Probe Support") -> ()
            n131 = global write "Collision Detection global.vi" "Model name"(w312) -> ()
          }
          frame #1 {
            n132 = property on="X Component" class="Ring (strict)"() -> ("Strings []"=w315:string[])  [unwired: 2 in, 2 out]
            n133 = Index Array(array=w315, index="X Component") -> (element=w314:string)
            n134 = local write "X string"(w314) -> ()
          }
          frame #2 {
            n135 = property on="XY Component (Traverse Boom)" class="Ring (strict)"() -> ("Strings []"=w319:string[])  [unwired: 2 in, 2 out]
            n136 = Index Array(array=w319, index="XY Component (Traverse Boom)") -> (element=w317:string)
            n137 = local write "XY string"(w317) -> ()
          }
          frame #3 {
            n138 = property on="XYZ Component (Measurement Probe)" class="Ring (strict)"() -> ("Strings []"=w322:string[])  [unwired: 2 in, 2 out]
            n139 = Index Array(array=w322, index="XYZ Component (Measurement Probe)") -> (element=w320:string)
            n140 = local write "XYZ string"(w320) -> ()
          }
          frame #4 {
            n141 = property on="Model Name" class="Ring (strict)"() -> ("Strings []"=w327:string[])  [unwired: 2 in, 2 out]
            n142 = Index Array(array=w327, index="Model Name") -> (element=w328:string)
            n143 = Not Equal?(x=w325, y=w328) -> (x != y?=w324:bool)
          }
          frame #5 {
            n144 = property on="Fixed Objects Name" class="Ring (strict)"() -> ("Strings []"=w330:string[])  [unwired: 2 in, 2 out]
            n145 = Index Array(array=w330, index="Fixed Objects Name") -> (element=w329:string)
          }
          frame #6 {
            n146 = property on="Traverse Name" class="Ring (strict)"() -> ("Strings []"=w338:string[])  [unwired: 2 in, 2 out]
            n147 = Index Array(array=w338, index="Traverse Name") -> (element=w336:string)
            n148 = Not Equal?(x=w337, y=w336) -> (x != y?=w335:bool)
            n149 = Compound Arithmetic op=OR(w332, "OK", w335) -> (w333:T3)
          }
        }
        n150 = Select(t=w303, s=w307, f="What to do next?") -> (s? t:f=w309:string)
        n151 = Select(t="Reset globals on Cancel", s=w306, f=w309) -> (s? t:f=w297:string)
        n152 = Select(t=w297, s=w299, f="Close Panel") -> (s? t:f=w296:string)
      }
      frame "Save Traverse limits" {
        n153 = local read "Traverse Limits"() -> (w344:T2)
        n154 = global write "Route_mapping_global.vi" "Traverse Limits"(w344) -> ()
        n155 = Equal?(x=w353, y=w344) -> (x = y?=w343:bool)
        n156 = case shown="False" w343 {
          tunnel: w348 -> [w358 _]
          tunnel: w347 -> [w357 _]
          tunnel: w346 -> [w356 _]
          tunnel: w345 -> [w355 _]
          tunnel: w344 -> [w354 _]
          frame False {
            n157 = Build Path(base path=w357, name or relative path=w358) -> (appended path=w360:path)
            n158 = Concatenate Strings(w358, w356) -> (w361:string)
            n159 = for {
              shift-right: [w370] -> w363
              shift-left: string[] [] -> [w372]
              tunnel: w354 -> [w367] mode=indexing
              n160 = Unbundle By Name(w367) -> ("Max"=w366:sgl, "Min"=w365:sgl)
              n161 = Max & Min(x=w366, y=w365) -> (max(x,y)=w369:sgl, min(x,y)=w368:sgl)
              n162 = Build Array(w369, w368) -> (w374:sgl[])
              n163 = Number To Fractional String(number=w374, precision (6)=i16 2) -> (F-format string=w371:string[])  [unwired: 2 out]
              n164 = Build Array (concatenate)(w372, w371) -> (w370:string[])
            }
            n165 = Build Path(base path=w360, name or relative path=w361) -> (appended path=w362:path)
            n166 = Build Array(w363) -> (w364:string[][])
            n167 = call "Write_Ch_data_file.vi"("Channel Values"=w364, "Channel names"=w355, "Filename"=w362) -> ()  [unwired: 4 in, 5 out]
          }
          frame True {
          }
        }
        n168 = global write "Route_mapping_global.vi" "Traverse Setup"(w348) -> ()
      }
      frame "Save Probe Support info" {
        n169 = local read "Probe Support"() -> (w380:T2)
        n170 = global write "Route_mapping_global.vi" "Probe Support"(w380) -> ()
        n171 = Equal?(x=w376, y=w380) -> (x = y?=w379:bool)
        n172 = case shown="False" w379 {
          tunnel: w383 -> [w392 _]
          tunnel: w382 -> [w391 _]
          tunnel: w377 -> [w390 _]
          tunnel: w381 -> [w389 _]
          tunnel: w380 -> [w388 _]
          frame False {
            n173 = Build Path(base path=w391, name or relative path=w392) -> (appended path=w394:path)
            n174 = Concatenate Strings(w392, w390) -> (w395:string)
            n175 = for {
              shift-right: [w404] -> w397
              shift-left: string[] [] -> [w406]
              tunnel: w388 -> [w401] mode=indexing
              n176 = Unbundle By Name(w401) -> ("Max"=w400:sgl, "Min"=w399:sgl)
              n177 = Max & Min(x=w400, y=w399) -> (max(x,y)=w403:sgl, min(x,y)=w402:sgl)
              n178 = Build Array(w403, w402) -> (w408:sgl[])
              n179 = Number To Fractional String(number=w408, precision (6)=i16 2) -> (F-format string=w405:string[])  [unwired: 2 out]
              n180 = Build Array (concatenate)(w406, w405) -> (w404:string[])
            }
            n181 = Build Path(base path=w394, name or relative path=w395) -> (appended path=w396:path)
            n182 = Build Array(w397) -> (w398:string[][])
            n183 = call "Write_Ch_data_file.vi"("Channel Values"=w398, "Channel names"=w389, "Filename"=w396) -> ()  [unwired: 4 in, 5 out]
          }
          frame True {
          }
        }
      }
      frame "Load another space file?" {
        n184 = stacked-sequence {
          seq-local: [w419 _] -> [_ w428]
          tunnel: w416 -> [w424 w426]
          tunnel: [w420 _] -> w415
          tunnel: [_ w431] -> w412
          tunnel: w414 -> [_ w430]
          tunnel: [_ w427] -> w413
          frame #0 {
            n185 = local read "Traverse Name"() -> (w418:u16)
            n186 = property on="Traverse Name" class="Ring (strict)"() -> ("Strings []"=w425:string[])  [unwired: 2 in, 2 out]
            n187 = Index Array(array=w425, index=w418) -> (element=w420:string)
            n188 = Not Equal?(x=w424, y=w420) -> (x != y?=w423:bool)
            n189 = Select(t="Get Traverse Names" ("f"), s=w423, f="Close Panel") -> (s? t:f=w419:string)
          }
          frame #1 {
            n190 = property on="Model Name" class="Ring (strict)"() -> ("Strings []"=w433:string[])  [unwired: 2 in, 2 out]
            n191 = local read "Model Name"() -> (w432:u16)
            n192 = Index Array(array=w433, index=w432) -> (element=w427:string)
            n193 = Not Equal?(x=w430, y=w427) -> (x != y?=w429:bool)
            n194 = case shown="True" w429 {
              tunnel: [w434 "Load Traverse Space info" ("f")] -> w431
              tunnel: w428 -> [w434 _]
              tunnel: w427 -> [_ w436]
              tunnel: w426 -> [_ w435]
              frame False {
              }
              frame True {
                n195 = call "Update_Selected_Space_File.vi"("Selected Space File Name"=w436, "Traverse Setup"=w435) -> ()  [unwired: 1 in]
              }
            }
          }
        }
      }
      frame "Reset globals on Cancel" {
        n196 = global write "Route_mapping_global.vi" "Traverse Setup"(w441) -> ()
        n197 = global write "Route_mapping_global.vi" "Traverse Limits"(w444) -> ()
        n198 = global write "Route_mapping_global.vi" "Probe Support"(w439) -> ()
        n199 = global write "Collision Detection global.vi" "Model name"(w440) -> ()
        n200 = global write "Collision Detection global.vi" "Fixed objects name"(w438) -> ()
      }
      frame "Close Panel" {
        n201 = call "Open_Close_Front_Panel.ph.vi"("openWindow (T)"=FALSE ("Front Panel Window:Open"), "VI path"=w478) -> ()  [unwired: 1 in, 1 out]
        n202 = Build Path(base path=w474, name or relative path=w463) -> (appended path=w462:path)
        n203 = Build Path(base path=w462, name or relative path=w464) -> (appended path=w475:path)
        n204 = local read "XYZ string"() -> (w467:string)
        n205 = Build Path(base path=w475, name or relative path=w459) -> (appended path=w447:path)
        n206 = Build Path(base path=w462, name or relative path=w461) -> (appended path=w460:path)
        n207 = Equal?(x=w456, y=w457) -> (x = y?=w458:bool)
        n208 = case shown="True" w458 {
          tunnel: w467 -> [w482 w485]
          tunnel: [w482 w484] -> w452
          frame False {
          }
          frame True {
            n209 = call "Mirror_Up_Down_Strings.vi"() -> ("Mirror Down"=w487:string, "Mirror Up"=w488:string)  [unwired: 2 in]
            n210 = global read "Trav_pos_global.vi" "Mirror Up?"() -> (w483:bool)
            n211 = Select(t=w488, s=w483, f=w487) -> (s? t:f=w486:string)
            n212 = Concatenate Strings(w485, w486) -> (w484:string)
          }
        }
        n213 = global read "Collision Detection global.vi" "X Components"() -> (w472:path)
        n214 = global read "Collision Detection global.vi" "XYZ Components"() -> (w469:path)
        n215 = global read "Collision Detection global.vi" "XY Components"() -> (w471:path)
        n216 = Build Path(base path=w460, name or relative path=w459) -> (appended path=w455:path)
        n217 = call "Write Characters with check.vi"("String to Write"=w454, "file (use dialog)"=w455) -> ()  [unwired: 2 in, 1 out]
        n218 = Strip Path(path=w472) -> (stripped path=w473:path)  [unwired: 1 out]
        n219 = Strip Path(path=w469) -> (stripped path=w466:path)  [unwired: 1 out]
        n220 = Strip Path(path=w471) -> (stripped path=w470:path)  [unwired: 1 out]
        n221 = call "Write Characters with check.vi"("String to Write"=w446, "file (use dialog)"=w447) -> ()  [unwired: 2 in, 1 out]
        n222 = Build Path(base path=w473, name or relative path=w459) -> (appended path=w448:path)
        n223 = Build Path(base path=w466, name or relative path=w459) -> (appended path=w453:path)
        n224 = Build Path(base path=w470, name or relative path=w459) -> (appended path=w451:path)
        n225 = local read "XY string"() -> (w450:string)
        n226 = local read "X string"() -> (w449:string)
        n227 = call "Write Characters with check.vi"("String to Write"=w452, "file (use dialog)"=w453) -> ()  [unwired: 2 in, 1 out]
        n228 = call "Write Characters with check.vi"("String to Write"=w449, "file (use dialog)"=w448) -> ()  [unwired: 2 in, 1 out]
        n229 = call "Write Characters with check.vi"("String to Write"=w450, "file (use dialog)"=w451) -> ()  [unwired: 2 in, 1 out]
        n230 = Build Path(base path=w466, name or relative path=w452) -> (appended path=w465:path)
        n231 = global write "Collision Detection global.vi" "XYZ Components"(w465) -> ()
      }
    }
  }
  n232 = global write "Collision Detection global.vi" "Force reload geometry"(TRUE ("Reload geometry")) -> ()
  "Error Comments" <- ""
